vi "Read Queue of Self Attributes.vi"(11 "Base Spawn in":refnum<class "Base Spawn.lvclass">) -> (2 "Queue of Self Attributes":refnum<queue>)   [LabVIEW 2025, in "jettl.lvlib" / "Spawn.lvlib" / "Base Spawn.lvclass"]
uses:
  Base Spawn.lvclass
  Base Spawn.lvclass/Base Spawn.ctl
  Attributes/Attributes/Attributes.lvclass
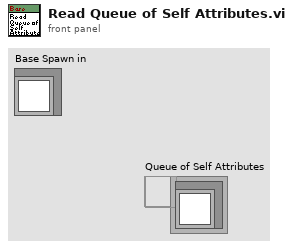
[diagram p1: front panel]
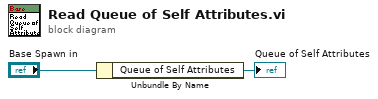
[diagram p0: block diagram]
diagram:
  n1 = Unbundle By Name("Base Spawn in") -> ("Queue of Self Attributes"=→"Queue of Self Attributes":refnum<queue>)
